vi "TSM Clear DAQmx Tasks.vi"(0 "TSM context":T1, 5 "Task Type":string[](array[string]), 7 "Reset recovery timeout (10s)":dbl=10.0) -> (15 "error out":errorcluster)   [LabVIEW 2020]
doc: "Use this VI to reset and clear all tasks for all NI-DAQmx instruments in the Semiconductor Module Context."
uses:
  <vilib>/NI_TestStand_SemiconductorModule/NI_TestStand_Semiconductor_Module.lvlibp/PinMap/General/SemiconductorModuleContext.ctl
  317af2ad-4c4f-4d56-a4e1-28ebb5a5f4d3.vi
  <vilib>/ErrorRing/Error Ring.xnode
  <vilib>/NI_TestStand_SemiconductorModule/NI_TestStand_Semiconductor_Module.lvlibp
  <resource>/objmgr/daqmx.rc
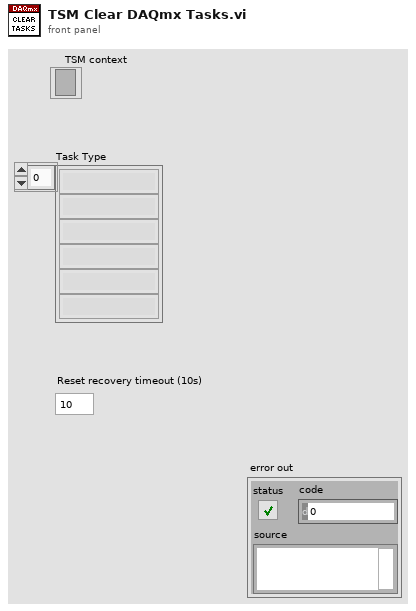
[diagram p1: front panel]
types:
  T1 = typedef "NI_TestStand_Semiconductor_Module.lvlibp/SemiconductorModuleContext.ctl" = refnum<k7>
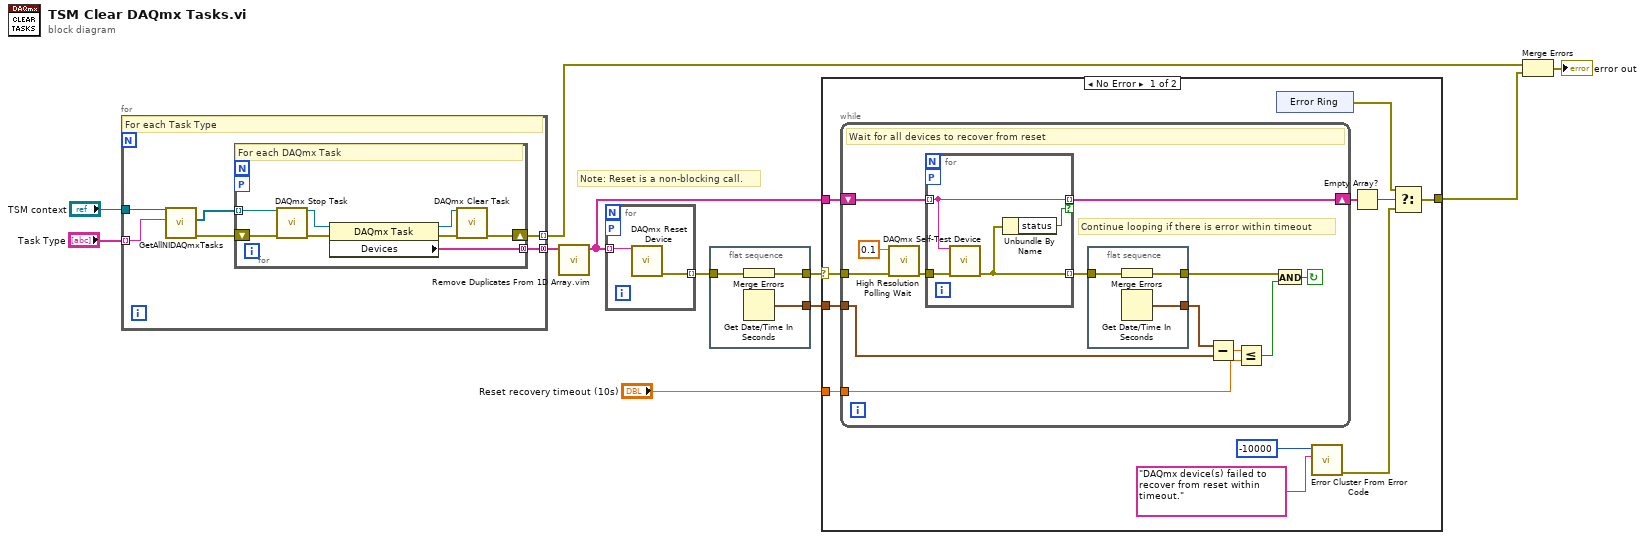
[diagram p0: block diagram]
diagram:
  # "Note: Reset is a non-blocking call."
  n1 = for {
    tunnel: [w16] -> w11 mode=indexing
    tunnel: "TSM context" -> [w14]
    tunnel: "Task Type" -> [w13] mode=indexing
    tunnel: [w12] -> w7 mode=concatenating
    # "For each Task Type"
    n2 = call <vilib>:"GetAllNIDAQmxTasks.vi"("Task Type"=w13, "Semiconductor Module Context"=w14) -> ("error out"=w15:errorcluster, "DAQmx Tasks"=w17:refnum<k21>[])  [unwired: 7 in, 1 out]
    n3 = for {
      tunnel: w17 -> [w24] mode=indexing
      shift-right: [w23] -> w16
      shift-left: w15 -> [w25]
      workers-P: _ -> [_]
      tunnel: [w18] -> w12 mode=concatenating
      # "For each DAQmx Task"
      n4 = call <vilib>:"DAQmx Stop Task.vi"("task/channels in"=w24, "error in"=w25) -> ("task out"=w20:refnum<k21>, "error out"=w22:errorcluster)  [unwired: 12 in]
      n5 = property class="DAQmx Task"(reference=w20, error in=w22) -> (reference out=w19:refnum<k21>, error out=w21:errorcluster, "Devices"=w18:tag[])
      n6 = call <vilib>:"DAQmx Clear Task.vi"("task in"=w19, "error in"=w21) -> ("error out"=w23:errorcluster)  [unwired: 13 in]
    }
  }
  n7 = call "Remove Duplicates From 1D Array.vim"("array"=w7) -> ("array with duplicates removed"=w6:tag[])  [unwired: 10 in]
  n8 = for {
    tunnel: w6 -> [w27] mode=indexing
    workers-P: _ -> [_]
    tunnel: [w26] -> w5 mode=indexing
    n9 = call <vilib>:"DAQmx Reset Device.vi"("device in"=w27) -> ("error out"=w26:errorcluster)  [unwired: 14 in]
  }
  n10 = flat-sequence {
    tunnel: w5 -> [w30]
    tunnel: [w28] -> w4
    tunnel: [w29] -> w3
    frame #0 {
      n11 = Merge Errors(w30) -> (w28:errorcluster)
      n12 = Get Date/Time In Seconds() -> (seconds since 1Jan1904=w29:timestamp)
    }
  }
  n13 = case shown="No Error" w4 {
    selector: w4 -> [w40 w63]
    tunnel: w6 -> [w41 _]
    tunnel: w3 -> [w39 _]
    tunnel: "Reset recovery timeout (10s)" -> [w38 _]
    tunnel: [w33 w63] -> w1
    frame No Error {
      n14 = while {
        tunnel: w40 -> [w54]
        tunnel: w39 -> [w49]
        tunnel: w38 -> [w44]
        shift-right: [w43] -> w32
        shift-left: w41 -> [w53]
        stop <- w47 continue-if-true
        # "Continue looping if there is error within timeout"
        # "Wait for all devices to recover from reset"
        n15 = call <vilib>:"High Resolution Polling Wait.vi"("error in (no error)"=w54, "seconds to wait"=0.1) -> ("error out"=w52:errorcluster)  [unwired: 9 in]
        n16 = for {
          tunnel: w52 -> [w61]
          tunnel: w53 -> [w60] mode=indexing
          workers-P: _ -> [_]
          tunnel: [w59] -> w42 mode=indexing
          tunnel: [w60] -> w43 mode=indexing if=w58
          n17 = call <vilib>:"DAQmx Self-Test Device.vi"("device in"=w60, "error in"=w61) -> ("error out"=w59:errorcluster)  [unwired: 13 in]
          n18 = Unbundle By Name(w59) -> ("status"=w58:bool)
        }
        n19 = flat-sequence {
          tunnel: w42 -> [w57]
          tunnel: [w55] -> w50
          tunnel: [w56] -> w48
          frame #0 {
            n20 = Merge Errors(w57) -> (w55:errorcluster)
            n21 = Get Date/Time In Seconds() -> (seconds since 1Jan1904=w56:timestamp)
          }
        }
        n22 = Subtract(x=w48, y=w49) -> (x-y=w46:dbl)
        n23 = Less Or Equal?(x=w46, y=w44) -> (x <= y?=w45:bool)
        n24 = And(x=w50, y=w45) -> (x .and. y?=w47:bool)
      }
      n25 = xnode "Error Ring"() -> ("error out"=w34:errorcluster)
      n26 = call <vilib>:"Error Cluster From Error Code.vi"("error message (\"\")"="DAQmx device(s) failed to recover from reset within timeout." ("format string"), "error code (0)"=-10000) -> ("error out"=w35:errorcluster)  [unwired: 7 in]
      n27 = Empty Array?(array=w32) -> (empty?=w31:bool)
      n28 = Select(t=w34, s=w31, f=w35) -> (s? t:f=w33:errorcluster)
    }
    frame Error {
      # "There was error in DAQmx reset"
    }
  }
  n29 = Merge Errors(w11, w1) -> (→"error out":errorcluster)
